vi "Refresh-display.vi"(8 "error in (no error)":errorcluster, 11 "Object ref in":T1) -> (0 "error out":errorcluster, 2 "Array":string[][](array[string]), 3 "Object ref out":T1)   [LabVIEW 2013, in "MaterialCharacterization.lvlib" / "MC-Main.lvclass"]
uses:
  MC-Main.lvclass
  Object-reference.ctl
  MC-Main.lvclass/MC-Main.ctl
  ScanParser/MC-ScanParser.lvclass/MC-ScanParser.ctl
  Read Parser.vi
  Read SM1000 positions.vi
  ScanParser/Read Path.vi
  ScanParser/MC-ScanParser.lvclass
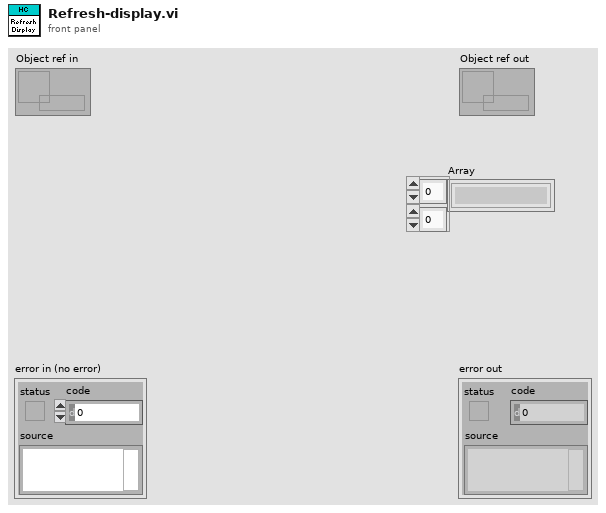
[diagram p1: front panel]
types:
  T1 = typedef "MaterialCharacterization.lvlib/MC-Main.lvclass/Object-reference.ctl" = refnum<data-value>
  T2 = typedef "MaterialCharacterization.lvlib/MC-ScanParser.lvclass/Object-reference.ctl" = refnum<data-value>
  T3 = typedef "HardwareCharacterization.lvlib/HC-ScanParser.lvclass/Point-buffer.ctl" = cluster{"Start time [µs]":i64, "End time [µs]":i64, "X [mm]":dbl, "Y [mm]":dbl, "Type":T4, "Speed [mm/µs]":dbl, "Direction [rad]":dbl, "X [bit]":i16, "Y [bit]":i16, "Speed [bit/µs]":dbl, "Power [W]":dbl, "Power [bit]":u8, "JumpDelay":i64, "MarkDelay":i64, "PolyDelay":i64, "LaserOnDelay":i64, "LaserOffDelay":i64, "LaserPowerDelay":i64, "LaserEnableDelay":i64, "Xraw [mm]":dbl, "Yraw [mm]":dbl}
  T4 = typedef "HardwareCharacterization.lvlib/Element-XML.lvclass/Elements.ctl" = enum16{"BeginJob", "WriteDigital", "WriteAnalog", "Set", "ApplicationEvent", "JumpAbs", "MarkAbs", "JumpRel", "MarkRel", "LongDelay", "EndJob"}
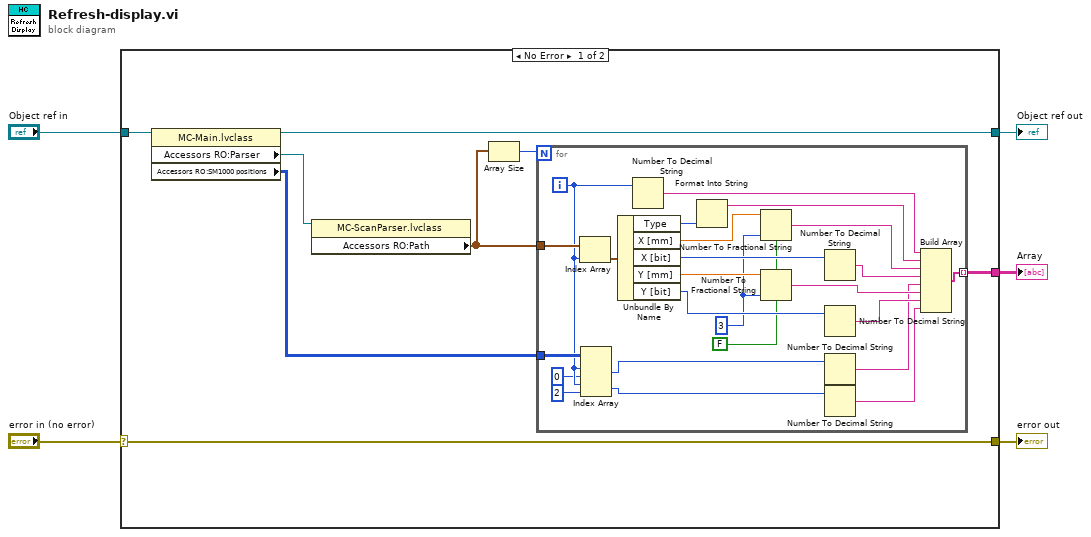
[diagram p0: block diagram]
diagram:
  n1 = case shown="No Error" "error in (no error)" {
    selector: "error in (no error)" -> [w13 w39]
    tunnel: [w13 w39] -> w4
    tunnel: [w11 w38] -> w2
    tunnel: "Object ref in" -> [w12 w38]
    tunnel: [w9 _] -> w1
    frame No Error {
      n2 = property class="MC-Main.lvclass"(reference=w12) -> (reference out=w11:T1, "Accessors RO:Parser"=w10:T2, "Accessors RO:SM1000 positions"=w6:i16[][])  [unwired: 1 in, 1 out]
      n3 = property class="MC-ScanParser.lvclass"(reference=w10) -> ("Accessors RO:Path"=w7:T3[])  [unwired: 1 in, 2 out]
      n4 = Array Size(array=w7) -> (size(s)=w8:i32)
      n5 = for {
        N: w8 -> [_]
        tunnel: w7 -> [w23]
        tunnel: [w24] -> w9 mode=indexing
        tunnel: w6 -> [w21]
        i -> [w20]
        w28 = FALSE ("use system decimal point (T)")
        w25 = i16 3 ("precision (6)")
        n6 = Index Array(array=w23, index=w20) -> (element=w22:T3)
        n7 = Index Array(array=w21, index (row) #1=w20, index (col) #1=0 ("disabled index (col)"), index (row) #2=w20, index (col) #2=2 ("disabled index (col)")) -> (element #1=w19:i16, element #2=w16:i16)
        n8 = Unbundle By Name(w22) -> ("Type"=w36:T4, "X [mm]"=w30:dbl, "X [bit]"=w34:i16, "Y [mm]"=w27:dbl, "Y [bit]"=w32:i16)
        n9 = Number To Decimal String(number=w20) -> (decimal integer string=w37:string)  [unwired: 1 in]
        n10 = Format Into String(w36) -> (resulting string=w35:string)  [unwired: 3 in, 1 out]
        n11 = Number To Fractional String(use system decimal point (T)=w28, number=w30, precision (6)=w25) -> (F-format string=w29:string)  [unwired: 1 in]
        n12 = Number To Fractional String(use system decimal point (T)=w28, number=w27, precision (6)=w25) -> (F-format string=w26:string)  [unwired: 1 in]
        n13 = Number To Decimal String(number=w34) -> (decimal integer string=w33:string)  [unwired: 1 in]
        n14 = Number To Decimal String(number=w32) -> (decimal integer string=w31:string)  [unwired: 1 in]
        n15 = Number To Decimal String(number=w19) -> (decimal integer string=w15:string)  [unwired: 1 in]
        n16 = Number To Decimal String(number=w16) -> (decimal integer string=w14:string)  [unwired: 1 in]
        n17 = Build Array(w37, w35, w29, w33, w15, w26, w31, w14) -> (w24:string[])
      }
    }
    frame Error {
    }
  }
  "error out" <- w4
  "Object ref out" <- w2
  "Array" <- w1
